vi "Gen3_L2_AiP_2x2_Mapping_20250125.vi"(7 "AiP":T1=1 items=["AiP_1"=1, "AiP_2"=2, "AiP_3"=3, "AiP_4"=4, "AiP_5"=5, "AiP_6"=6, "AiP_7"=7, "AiP_8"=8, "AiP_9"=9, "AiP_10"=10, "AiP_11"=11, "AiP_12"=12, "AiP_13"=13, "AiP_14"=14, "AiP_15"=15, "AiP_16"=16]) -> (1 "Pol_V":i32[](array[numeric]), 2 "Pol_H":i32[](array[numeric]), 3 "Ch_Index":i32[](array[numeric]))   [LabVIEW 2023]
uses:
  CTL/AiP_index.ctl
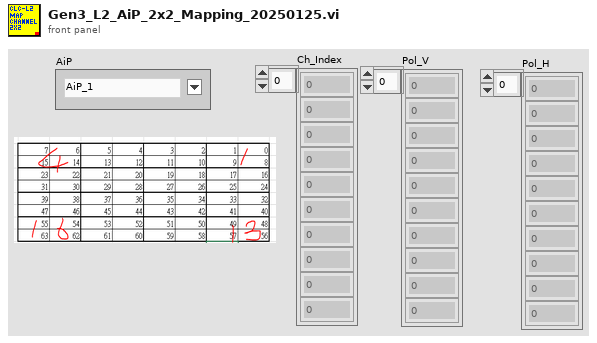
[diagram p1: front panel]
types:
  T1 = typedef "AiP_index.ctl" = u16
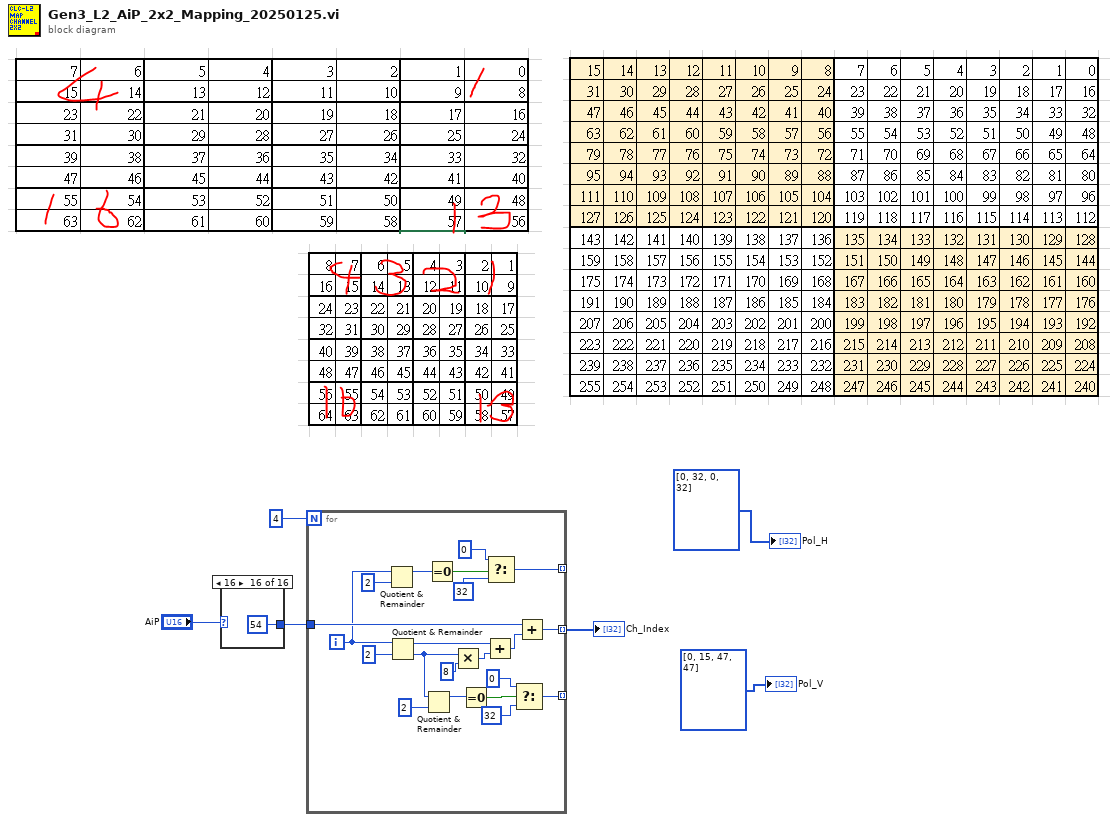
[diagram p0: block diagram]
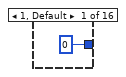
[diagram p2: hidden frame]
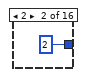
[diagram p3: hidden frame]
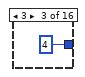
[diagram p4: hidden frame]
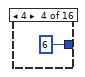
[diagram p5: hidden frame]
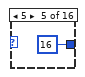
[diagram p6: hidden frame]
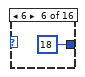
[diagram p7: hidden frame]
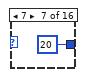
[diagram p8: hidden frame]
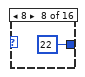
[diagram p9: hidden frame]
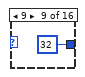
[diagram p10: hidden frame]
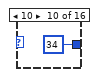
[diagram p11: hidden frame]
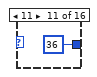
[diagram p12: hidden frame]
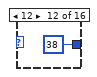
[diagram p13: hidden frame]
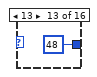
[diagram p14: hidden frame]
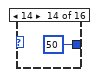
[diagram p15: hidden frame]
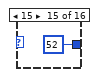
[diagram p16: hidden frame]
diagram:
  n1 = case shown="16" "AiP" {
    tunnel: [0 ("y") 2 ("y") 4 ("y") 6 ("y") 16 ("y") 18 ("y") 20 ("y") 22 ("y") 32 ("y") 34 ("y") 36 ("y") 38 ("y") 48 ("y") 50 ("y") 52 ("y") 54 ("y")] -> w3
    frame 1, Default {
    }
    frame 2 {
    }
    frame 3 {
    }
    frame 4 {
    }
    frame 5 {
    }
    frame 6 {
    }
    frame 7 {
    }
    frame 8 {
    }
    frame 9 {
    }
    frame 10 {
    }
    frame 11 {
    }
    frame 12 {
    }
    frame 13 {
    }
    frame 14 {
    }
    frame 15 {
    }
    frame 16 {
    }
  }
  n2 = for {
    N: 4 -> [_]
    tunnel: [w38] -> w5 mode=indexing
    tunnel: w3 -> [w39]
    tunnel: [w33] -> _ mode=indexing
    tunnel: [w23] -> _ mode=indexing
    i -> [w32]
    n3 = Quotient & Remainder(x=w32, y=2) -> (x-y*floor(x/y)=w30:i32)  [unwired: 1 out]
    n4 = Quotient & Remainder(x=w32, y=2) -> (x-y*floor(x/y)=w37:i32, floor(x/y)=w28:i32)
    n5 = Quotient & Remainder(x=w28, y=2) -> (x-y*floor(x/y)=w25:i32)  [unwired: 1 out]
    n6 = Equal To 0?(x=w30) -> (x = 0?=w36:bool)
    n7 = Multiply(x=w28, y=8) -> (x*y=w41:i32)
    n8 = Equal To 0?(x=w25) -> (x = 0?=w24:bool)
    n9 = Add(x=w37, y=w41) -> (x+y=w40:i32)
    n10 = Select(t=0 ("Phase"), s=w36, f=32 ("Phase")) -> (s? t:f=w33:i32)
    n11 = Select(t=0 ("Phase"), s=w24, f=32 ("Phase")) -> (s? t:f=w23:i32)
    n12 = Add(x=w39, y=w40) -> (x+y=w38:i32)
  }
  "Ch_Index" <- w5
  "Pol_V" <- i32[] [0, 15, 47, 47] ("Pol_H")
  "Pol_H" <- i32[] [0, 32, 0, 32] ("Pol_H")
